vi "Abort Test.vi"(7 "abort test?":bool, 8 "error in (no error)":errorcluster, 9 "time (sec)":dbl, 10 "diameter (mm)":dbl, 11 "IA Test Parameters in":refnum<class "IA Test Parameters.lvclass">) -> (0 "error out":errorcluster, 3 "test aborted?":bool)   [LabVIEW 2020]
uses:
  Parameter Class/IA Test Parameters.lvclass
  Parameter Class/IA Test Parameters.lvclass/IA Test Parameters.ctl
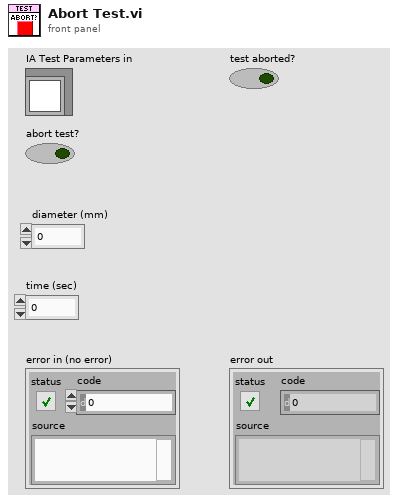
[diagram p1: front panel]
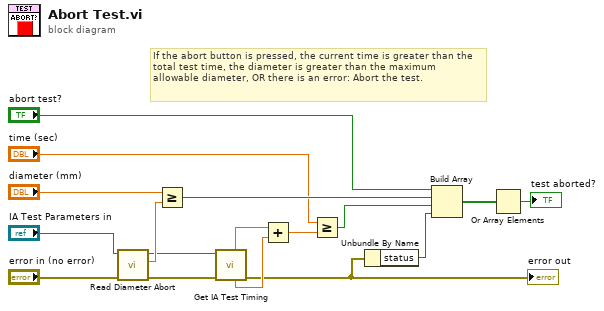
[diagram p0: block diagram]
diagram:
  # "If the abort button is pressed, the current time is greater than the total test time, the diameter is greater than the maximum allowable diameter, OR there is an error: Abort the test."
  n1 = call "Read Diameter Abort.vi"("error in (no error)"="error in (no error)", "IA Test Parameters in"="IA Test Parameters in") -> ("error out"=w2:errorcluster, "diameter abort (mm)"=w16:dbl, "IA Test Parameters out"=w4:refnum<class "IA Test Parameters.lvclass">)  [unwired: 7 in]
  n2 = Greater Or Equal?(x="diameter (mm)", y=w16) -> (x >= y?=w14:bool)
  n3 = call "Get IA Test Timing.vi"("error in (no error)"=w2, "IA Test Parameters in"=w4) -> ("error out"=w1:errorcluster, "test time (sec)"=w11:dbl, "time delay (sec)"=w12:dbl)  [unwired: 4 in, 3 out]
  "error out" <- w1
  n4 = Add(x=w12, y=w11) -> (x+y=w10:dbl)
  n5 = Greater Or Equal?(x="time (sec)", y=w10) -> (x >= y?=w6:bool)
  n6 = Unbundle By Name(w1) -> ("status"=w13:bool)
  n7 = Build Array("abort test?", w14, w6, w13) -> (w7:bool[])
  n8 = Or Array Elements(Boolean array=w7) -> (logical OR=→"test aborted?":bool)
